vi "mfd_get.vi"(7 "MFD_Stop":bool) -> (20 "MFD_StatusText":picture, 21 "MFD_RadioBattery":picture, 22 "MFD_Gps":picture)   [LabVIEW 2023]
uses:
  mfd_global.vi
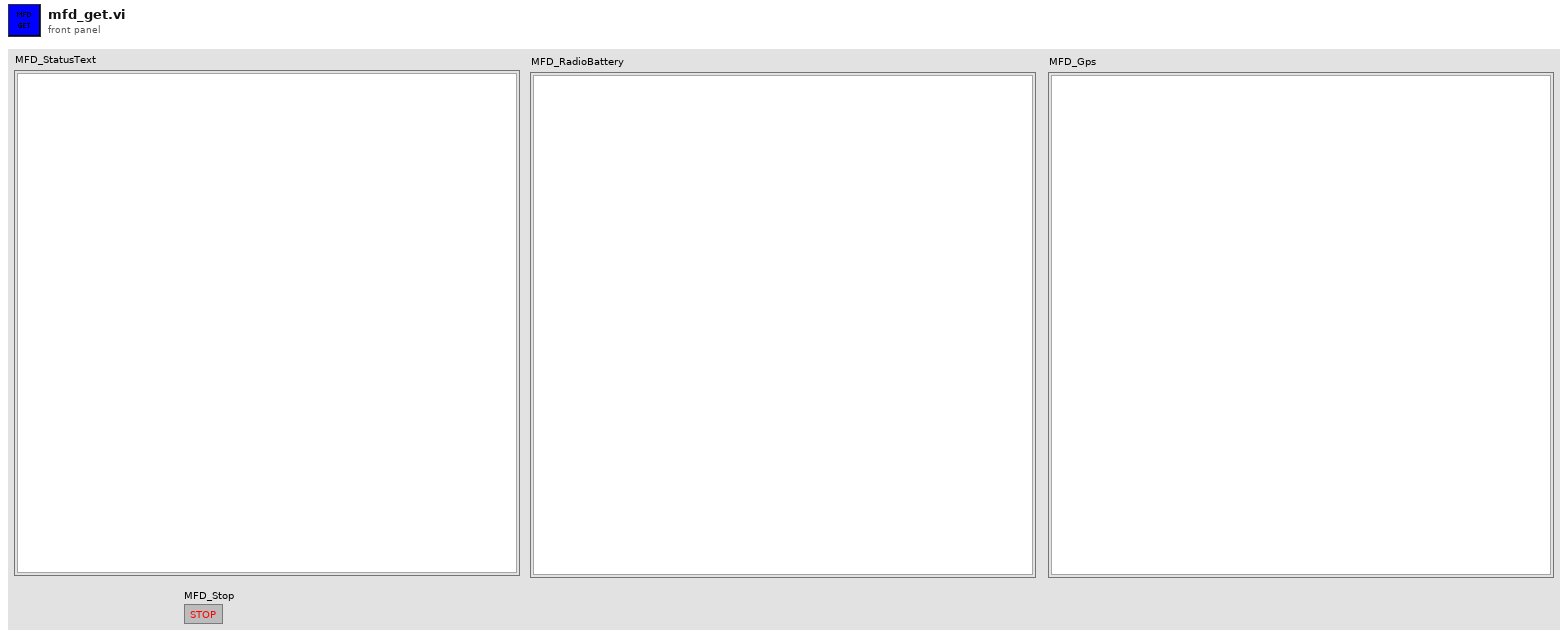
[diagram p1: front panel]
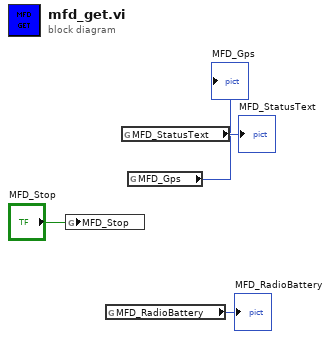
[diagram p0: block diagram]
diagram:
  n1 = global write "mfd_global.vi" "MFD_Stop"("MFD_Stop") -> ()
  n2 = global read "mfd_global.vi" "MFD_RadioBattery"() -> (→"MFD_RadioBattery":picture)
  n3 = global read "mfd_global.vi" "MFD_StatusText"() -> (→"MFD_StatusText":picture)
  n4 = global read "mfd_global.vi" "MFD_Gps"() -> (→"MFD_Gps":picture)
